vi "AB Command Voltage Limit.vi"(9 "Max Voltage":dbl, 11 "Command In":dbl) -> (2 "Command Out":dbl)   [LabVIEW 2013]
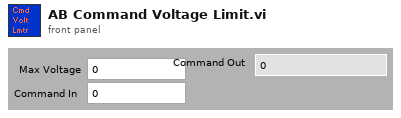
[diagram p1: front panel]
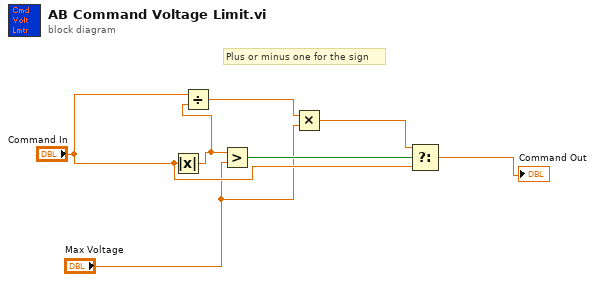
[diagram p0: block diagram]
diagram:
  # "Plus or minus one for the sign"
  n1 = Absolute Value(x="Command In") -> (abs(x)=w7:dbl)
  n2 = Divide(x="Command In", y=w7) -> (x/y=w4:dbl)
  n3 = Greater?(x=w7, y="Max Voltage") -> (0:w6:bool)
  n4 = Multiply(x=w4, y="Max Voltage") -> (x*y=w2:dbl)
  n5 = Select(t=w2, s=w6, f="Command In") -> (s? t:f=→"Command Out":dbl)
